vi "Master_EmergencyCheck.vi"(8 "CheckData in":refnum<class "CheckData.lvclass">[](array[class]), 10 "State in":T2, 11 "Actuators in":T1) -> (0 "CheckData out":refnum<class "CheckData.lvclass">[](array[class]), 2 "Fault?":bool)   [LabVIEW 2017]
doc: "Can be disabled from Host Front Panel control \"Disable ECheck\"\nCreates an array of objects of the CheckData class which holds a sensor value and its preset maximum and minimum vales to be considered \"safe\" or of normal operation."
uses:
  CheckData/CheckData.lvclass
  TypeDef_ControlState.ctl
  TypeDef_DigitalOuts.ctl
  DAQ/Master_DataControl.ctl
  DAQ/TypeDef_cRIOData.ctl
  IMU/TypeDef_IMUData.ctl
  CAN/TypeDef_BMSData.ctl
  CAN/TypeDef_BMS_Status.ctl
  CAN/MotorController/fixedMotorData.ctl
  CAN/MotorController/MotorStatus.ctl
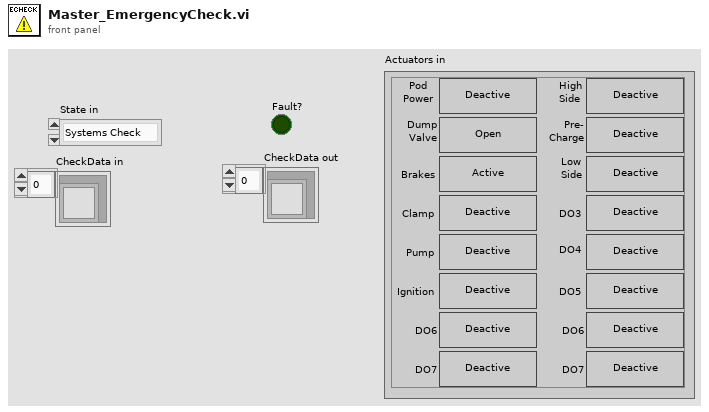
[diagram p1: front panel]
types:
  T1 = typedef "TypeDef_DigitalOuts.ctl" = cluster{"Pod Power":bool, "Dump Valve":bool, "Brakes":bool, "Clamp":bool, "Pump":bool, "Ignition":bool, "DO6":bool, "DO7":bool, "HighSide":bool, "Precharge":bool, "LowSide":bool, "DO3":bool, "DO4":bool, "DO5":bool, "DO62":bool, "DO72":bool}
  T2 = typedef "TypeDef_ControlState.ctl" = enum16{"Systems Check", "Idle", "Ready", "Pushing", "Coast", "Braking", "Fault", "Shutdown", "Service", "Precharge", "Blank"}
  T3 = typedef "Master_DataControl.ctl" = cluster{"cRIO Data":T4, "IMU Data":T5, "BMS Data":T6, "Motor Data":T8}
  T4 = typedef "TypeDef_cRIOData.ctl" = cluster{"Time (ms)":dbl, "24V Battery (V)":dbl, "LowV Current (A)":dbl, "Fiducial Sensor (V)":dbl, "PV Pressure (psig)":dbl, "Flow Sensor (V)":dbl, "Temp Fairing (F)":dbl, "Temp Reservoir (F)":dbl, "HallEffect Right (in)":dbl, "HallEffect Left (in)":dbl, "PT Tank (psig)":dbl, "PT Clamp Right (psig)":dbl, "PT Clamp Left (psig)":dbl, "PT Brake (psig)":dbl, "PT Cooling (psig)":dbl, "Displacement (ft)":dbl, "Velocity (ft/s)":dbl}
  T5 = typedef "TypeDef_IMUData.ctl" = cluster{"x acceleration (g)":dbl, "Pressure (psia)":dbl, "Temperature (F)":dbl}
  T6 = typedef "TypeDef_BMSData.ctl" = cluster{"Max Cell Voltage (V)":dbl, "Max Cell ID":dbl, "Min Cell Voltage (V)":dbl, "Min Cell ID":dbl, "State of Charge (%)":dbl, "Average Voltage (V)":dbl, "Voltage Delta (V)":dbl, "Pack Current (A)":dbl, "Pack Voltage (V)":dbl, "Max Resistance (Ohm)":dbl, "Min Resistance (Ohm)":dbl, "Average Resistance (Ohm)":dbl, "Delta Resistance (Ohm)":dbl, "Highest Temperature(F)":dbl, "BmsStatus":T7}
  T7 = typedef "TypeDef_BMS_Status.ctl" = cluster{"isFault":bool, "isolationMonitoring":bool}
  T8 = typedef "fixedMotorData.ctl" = cluster{"Velo (RPM)":dbl, "MotorTemp(F)":dbl, "CtrlTemp(F)":dbl, "DcLinkVolt(V)":dbl, "ErrorCode":dbl, "motorStatus":T9, "isAlive":bool, "motorControllerState":u16}
  T9 = typedef "MotorStatus.ctl" = cluster{"isReady":bool, "isOn":bool, "isOperEn":bool, "isFault":bool, "isVoltEn":bool, "targetReached":bool, "isWarning":bool}
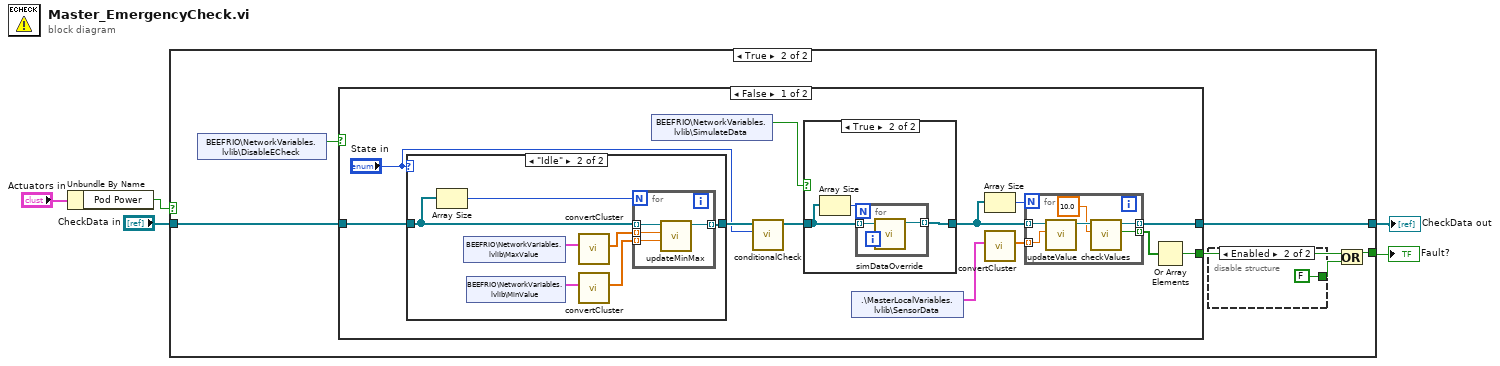
[diagram p0: block diagram]
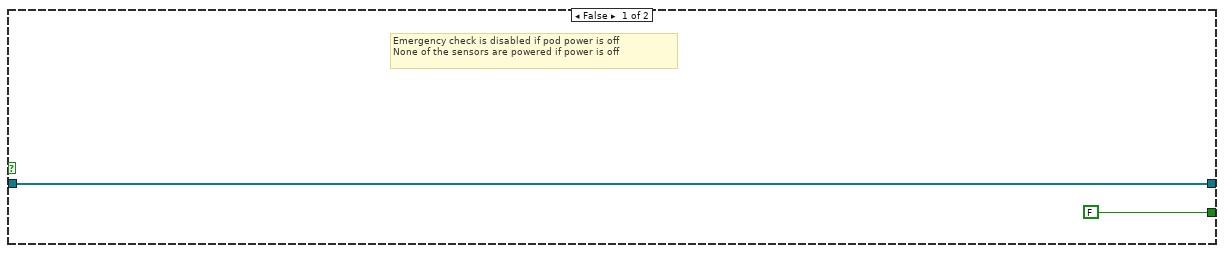
[diagram p2: hidden frame]
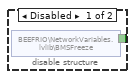
[diagram p3: hidden frame]
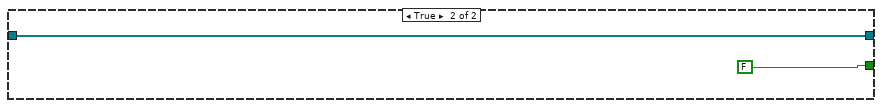
[diagram p6: hidden frame]
diagram:
  n1 = Unbundle By Name("Actuators in") -> ("Pod Power"=w3:bool)
  n2 = case shown="True" w3 {
    tunnel: [w6 w13] -> w5
    tunnel: [FALSE w9] -> w2
    tunnel: "CheckData in" -> [w6 w8]
    frame False {
      # "Emergency check is disabled if pod power is off\nNone of the sensors are powered if power is off"
    }
    frame True {
      n3 = shared-variable "BEEFRIO\\NetworkVariables.lvlib\\DisableECheck"() -> (w12:bool)  [unwired: 1 in, 1 out]
      n4 = case shown="False" w12 {
        tunnel: [w23 w53] -> w13
        tunnel: w8 -> [w22 w53]
        tunnel: [w21 FALSE] -> w10
        frame False {
          n5 = case shown="\"Idle\"" "State in" {
            tunnel: w22 -> [w34 w39]
            tunnel: [w34 w41] -> w20
            frame Default {
            }
            frame "Idle" {
              n6 = Array Size(array=w39) -> (size(s)=w40:i32)
              n7 = shared-variable "BEEFRIO\\NetworkVariables.lvlib\\MaxValue"() -> (w37:T3)  [unwired: 1 in, 1 out]
              n8 = shared-variable "BEEFRIO\\NetworkVariables.lvlib\\MinValue"() -> (w38:T3)  [unwired: 1 in, 1 out]
              n9 = call "convertCluster.vi"("Data"=w37) -> ("Array"=w36:dbl[])  [unwired: 10 in]
              n10 = call "convertCluster.vi"("Data"=w38) -> ("Array"=w35:dbl[])  [unwired: 10 in]
              n11 = for {
                N: w40 -> [_]
                tunnel: [w45] -> w41 mode=indexing
                tunnel: w39 -> [w44] mode=indexing
                tunnel: w36 -> [w43] mode=indexing
                tunnel: w35 -> [w42] mode=indexing
                n12 = call "updateMinMax.vi"("Min Value"=w42, "Max Value"=w43, "CheckData in"=w44) -> ("CheckData out"=w45:refnum<class "CheckData.lvclass">)  [unwired: 8 in]
              }
            }
          }
          n13 = shared-variable "BEEFRIO\\NetworkVariables.lvlib\\SimulateData"() -> (w16:bool)  [unwired: 1 in, 1 out]
          n14 = call "conditionalCheck.vi"("State in"="State in", "CheckData in in"=w20) -> ("CheckData out"=w18:refnum<class "CheckData.lvclass">[])  [unwired: 9 in]
          n15 = case shown="True" w16 {
            tunnel: w18 -> [w28 w30]
            tunnel: [w28 w29] -> w17
            frame False {
            }
            frame True {
              n16 = Array Size(array=w30) -> (size(s)=w31:i32)
              n17 = for {
                N: w31 -> [_]
                tunnel: w30 -> [w33] mode=indexing
                tunnel: [w32] -> w29 mode=indexing
                n18 = call "simDataOverride.vi"("CheckData in"=w33) -> ("CheckData out"=w32:refnum<class "CheckData.lvclass">)  [unwired: 10 in]
              }
            }
          }
          n19 = shared-variable ".\\MasterLocalVariables.lvlib\\SensorData"() -> (w24:T3)  [unwired: 1 in, 1 out]
          n20 = Array Size(array=w17) -> (size(s)=w27:i32)
          n21 = call "convertCluster.vi"("Data"=w24) -> ("Array"=w26:dbl[])  [unwired: 10 in]
          n22 = for {
            N: w27 -> [_]
            tunnel: w17 -> [w51] mode=indexing
            tunnel: w26 -> [w50] mode=indexing
            tunnel: [w48] -> w23 mode=indexing
            tunnel: [w47] -> w25 mode=indexing
            n23 = call "updateValue.vi"("Current Value in"=w50, "CheckData in"=w51) -> ("CheckData out"=w49:refnum<class "CheckData.lvclass">)  [unwired: 9 in]
            n24 = call "checkValues.vi"("Threshold"=10.0, "CheckData in"=w49) -> ("Fault"=w47:bool, "CheckData out"=w48:refnum<class "CheckData.lvclass">)  [unwired: 8 in]
          }
          n25 = Or Array Elements(Boolean array=w25) -> (logical OR=w21:bool)
        }
        frame True {
        }
      }
      n26 = disable-structure shown="Enabled" {
        disable-tunnel: [w14 FALSE] -> w11
        frame Disabled {
          n27 = shared-variable "BEEFRIO\\NetworkVariables.lvlib\\BMSFreeze"() -> (w14:bool)  [unwired: 1 in, 1 out]
        }
        frame Enabled {
        }
      }
      n28 = Or(x=w10, y=w11) -> (x .or. y?=w9:bool)
    }
  }
  "CheckData out" <- w5
  "Fault?" <- w2
